vi "JSONError.vi"(9 "error":string) -> (3 "JSON string":string)   [LabVIEW 2026]
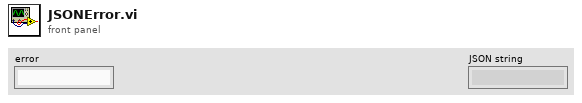
[diagram p1: front panel]
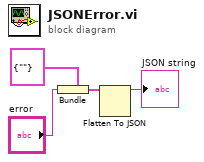
[diagram p0: block diagram]
diagram:
  n1 = Bundle(cluster=cluster{"error":string} {"error"=""}, "error"="error") -> (w4:cluster{"error":string})
  n2 = Flatten To JSON(anything=w4) -> (JSON string=→"JSON string":string)  [unwired: 2 in, 1 out]
